vi "myread.vi"(8 "Boolean":bool, 11 "Network":T1={"invert_send"=TRUE, "Number of datagrams to read"=5000, "max bytes/read"=2500, "Timeout"=4000, "host"="192.168.1.18", "Port Receive"=5678} {"Number of datagrams to read" format="%0d"}) -> ()   [LabVIEW 2014]
uses:
  controls/Network.ctl
panel:
  out "data out":string
  in  "error in (no error)":errorcluster
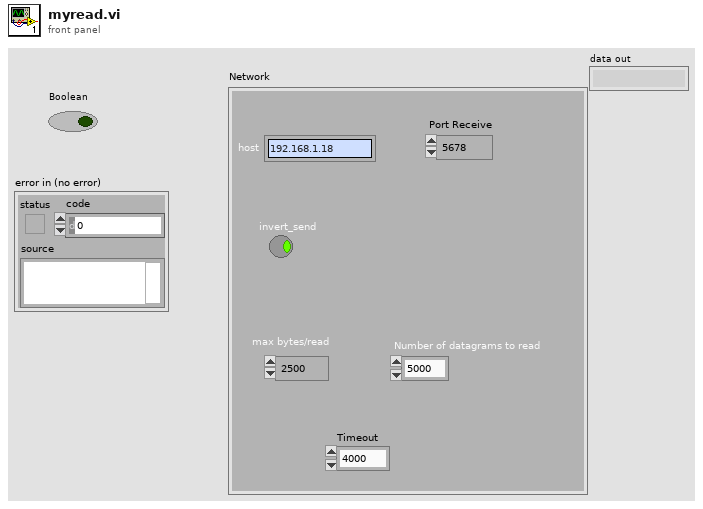
[diagram p1: front panel]
types:
  T1 = typedef "Network.ctl" = cluster{"invert_send":bool, "Number of datagrams to read":u32, "max bytes/read":i32, "Timeout":i32, "host":string, "Port Receive":u16}
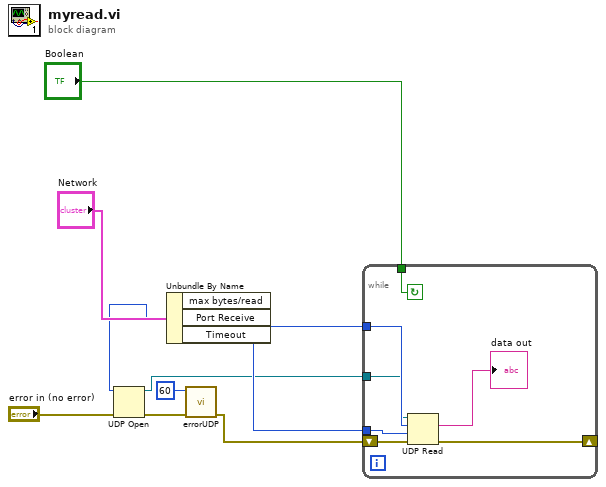
[diagram p0: block diagram]
diagram:
  n1 = Unbundle By Name("Network") -> ("max bytes/read"=w5:i32, "Port Receive"=w6:u16, "Timeout"=w4:i32)
  n2 = UDP Open(8:"error in (no error)", 11:w6) -> (port=w1:refnum<k16>, 0:w9:errorcluster)  [unwired: 4 out]
  n3 = call "errorUDP.vi"("error in (no error) 2"=w9, "errorcode"=60) -> ("error out 2"=w3:errorcluster)  [unwired: 9 out]
  n4 = while {
    shift-right: [w16] -> _
    shift-left: w3 -> [w17]
    tunnel: w5 -> [w15]
    tunnel: w4 -> [w14]
    tunnel: "Boolean" -> [w12]
    tunnel: w1 -> [w11]
    stop <- w12 continue-if-true
    n5 = UDP Read(connection ID=w11, max size (548)=w15, timeout ms (25000)=w14, 8:w17) -> (data out=→"data out":string, error out=w16:errorcluster)  [unwired: 3 out]
  }
